vi "dequeue_command_by_dim_name.vi"(8 "error in (no error)":errorcluster caption="错误输入（无错误）", 10 "name":string, 11 "MotorSystem 输入":refnum<class "MotorSystem.lvclass">) -> (0 "error out":errorcluster caption="错误输出", 2 "command":cluster{"cmd":T1, "cmd data":variant}, 3 "MotorSystem 输出":refnum<class "MotorSystem.lvclass">)   [LabVIEW 2016, in "MotionControl.lvlib" / "MotorSystem.lvclass"]
uses:
  <userlib>/MotionControl/MotorSystem/MotorSystem.lvclass
  <userlib>/MotionControl/OneMotion/cmd_motion.ctl
  <userlib>/MotionControl/MotorSystem/MotorSystem.lvclass/MotorSystem.ctl
  <userlib>/MotionControl/OneMotion/OneMotion.lvclass
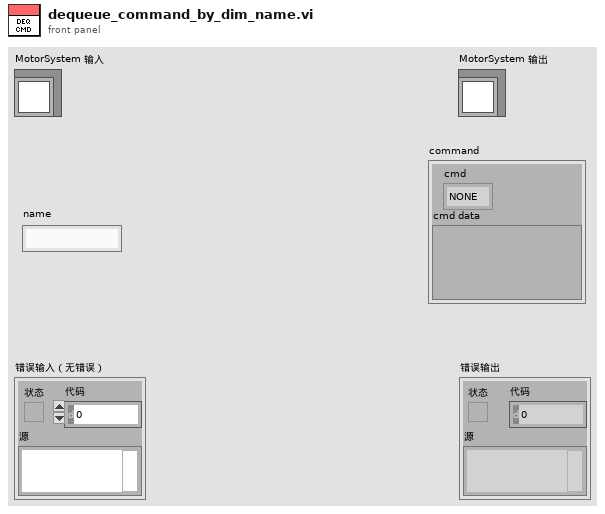
[diagram p1: front panel]
types:
  T1 = typedef "MotionControl.lvlib/OneMotion.lvclass/cmd_motion.ctl" = enum16{"NONE", "MOVE_MOTION", "EXIT", "STP_MOTION", "SPEED_MOTION", "WAIT_FOR_S3", "WAIT_A_TIME", "SKIP"}
  T2 = typedef "MotionControl.lvlib/MotorSystem.lvclass/MotionCluster.ctl" = cluster{"OneMotion.lvclass":refnum<class "OneMotion.lvclass">, "connected?":bool, "default enabled?":bool, "enabled?":bool}
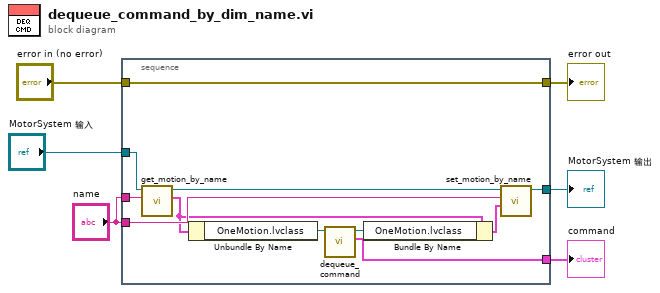
[diagram p0: block diagram]
diagram:
  n1 = stacked-sequence {
    tunnel: [w7] -> w6
    tunnel: [w9] -> w4
    tunnel: "MotorSystem 输入" -> [w17]
    tunnel: "name" -> [w16]
    tunnel: "name" -> [w14]
    tunnel: [w8] -> w2
    tunnel: "error in (no error)" -> [w7]
    frame #0 {
      n2 = call <userlib>:"get_motion_by_name.vi"("name"=w16, "MotorSystem in"=w17) -> ("motion cluster"=w12:T2, "MotorSystem out"=w13:refnum<class "MotorSystem.lvclass">)  [unwired: 7 in, 1 out]
      n3 = Unbundle By Name(w12) -> ("OneMotion.lvclass"=w15:refnum<class "OneMotion.lvclass">)
      n4 = call <userlib>:"dequeue_command.vi"("OneMotion输入"=w15) -> ("command"=w8:cluster{"cmd":T1, "cmd data":variant}, "OneMotion输出"=w11:refnum<class "OneMotion.lvclass">)  [unwired: 8 in, 1 out]
      n5 = Bundle By Name(cluster=w12, "OneMotion.lvclass"=w11) -> (w10:T2)
      n6 = call <userlib>:"set_motion_by_name.vi"("簇"=w10, "name"=w14, "MotorSystem输入"=w13) -> ("MotorSystem输出"=w9:refnum<class "MotorSystem.lvclass">)  [unwired: 7 in, 1 out]
    }
  }
  "error out" <- w6
  "MotorSystem 输出" <- w4
  "command" <- w2
